vi "Compensate For Hit Position.vi"(8 "Primary channel":i8, 9 "Secondary hit time":u64, 10 "Secondary channel":i8, 11 "Primary hit time":u64) -> (2 "Secondary true hit time":u64, 3 "Primary true hit time":u64)   [LabVIEW 2016]
uses:
  Global Variables/Global Resolution.vi
panel:
  # "Calculates the actual muon hit time by compensating for the time it takes the photons to reach the SiPM"
  # "Leave primary hit time unwired to calculate secondary hit time and vice versa"
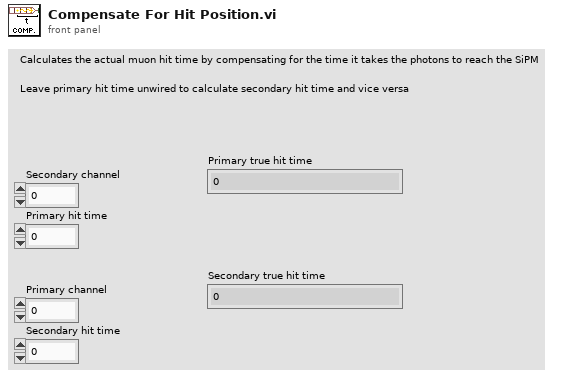
[diagram p1: front panel]
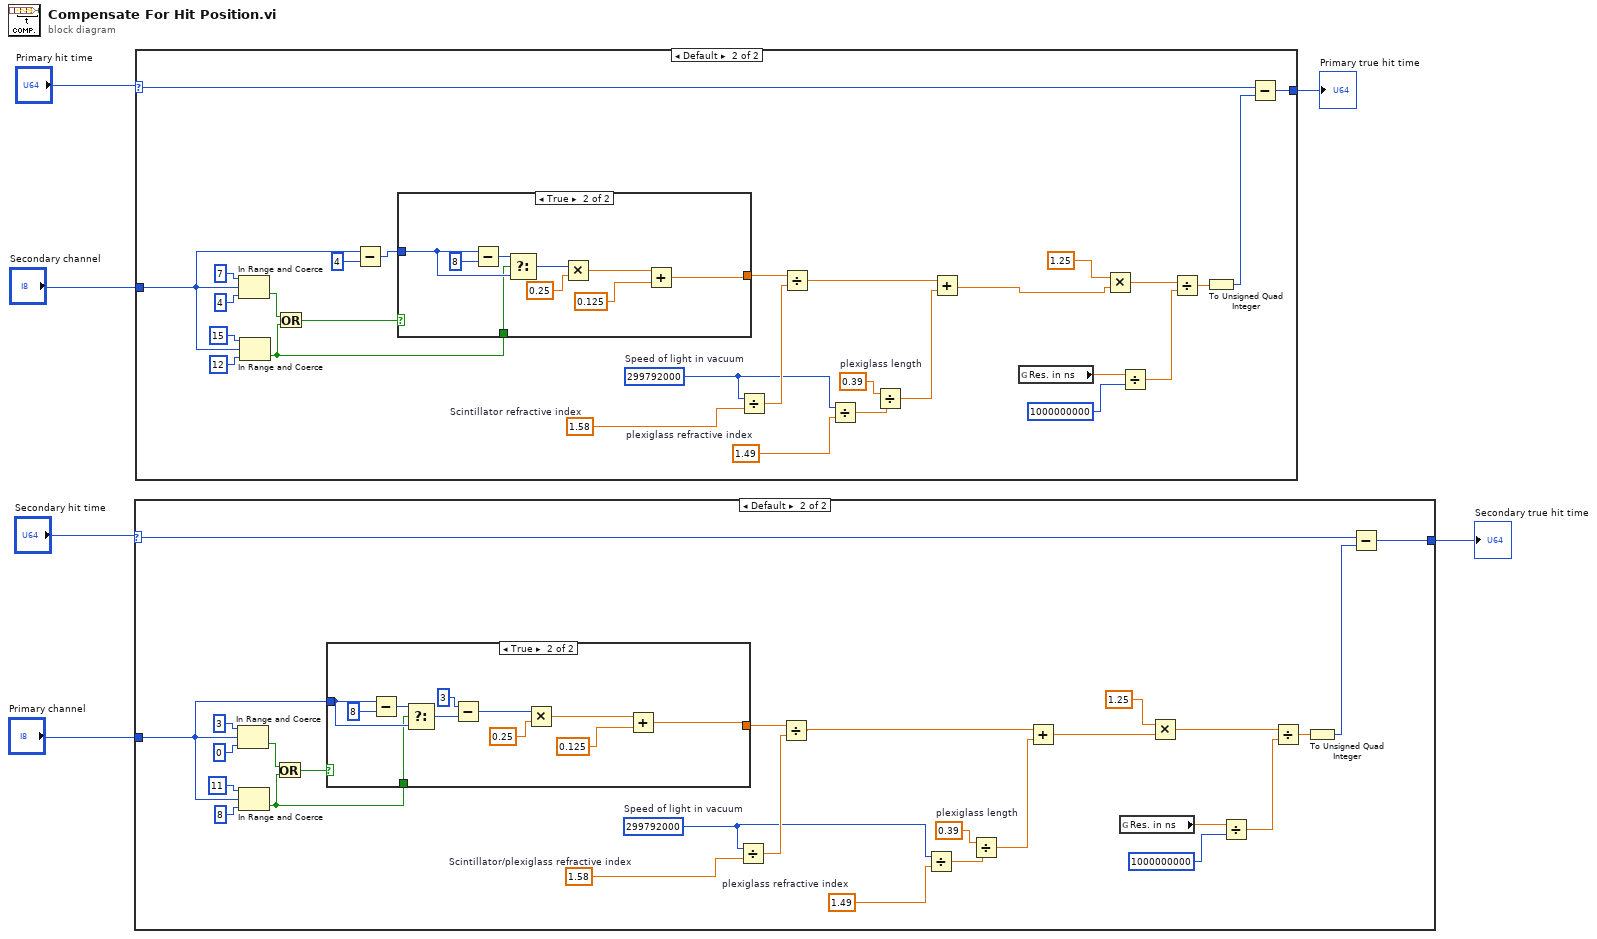
[diagram p0: block diagram]
diagram:
  n1 = case shown="Default" "Secondary hit time" {
    selector: "Secondary hit time" -> [w7 w18]
    tunnel: [w7 w19] -> w1
    tunnel: "Primary channel" -> [_ w17]
    frame 0 {
    }
    frame Default {
      w15 = 0.39  # plexiglass length
      w16 = 1.49  # plexiglass refractive index
      w11 = 299792000  # Speed of light in vacuum
      w34 = 1.58  # Scintillator/plexiglass refractive index
      n2 = In Range and Coerce(upper limit=3, x=w17, lower limit=0) -> (In Range?=w28:bool)  [unwired: 1 out]
      n3 = In Range and Coerce(upper limit=11, x=w17, lower limit=8) -> (In Range?=w27:bool)  [unwired: 1 out]
      n4 = Or(x=w28, y=w27) -> (x .or. y?=w29:bool)
      n5 = case shown="True" w29 {
        tunnel: w17 -> [_ w43]
        tunnel: w27 -> [_ w42]
        tunnel: [_ w35] -> w26
        frame False {
        }
        frame True {
          n6 = Subtract(x=w43, y=8) -> (x-y=w44:i32)
          n7 = Select(t=w44, s=w42, f=w43) -> (s? t:f=w38:i32)
          n8 = Subtract(x=3 ("y"), y=w38) -> (x-y=w40:i32)
          n9 = Multiply(x=w40, y=0.25) -> (x*y=w36:dbl)
          n10 = Add(x=w36, y=0.125) -> (x+y=w35:dbl)
        }
      }
      n11 = Divide(x=w11, y=w34) -> (x/y=w25:dbl)
      n12 = Divide(x=w26, y=w25) -> (x/y=w12:dbl)
      n13 = Divide(x=w11, y=w16) -> (x/y=w14:dbl)
      n14 = Divide(x=w15, y=w14) -> (x/y=w13:dbl)
      n15 = Add(x=w12, y=w13) -> (x+y=w10:dbl)
      n16 = global read "Global Resolution.vi" "Res. in ns"() -> (w22:ext)
      n17 = Multiply(x=1.25, y=w10) -> (x*y=w9:dbl)
      n18 = Divide(x=w22, y=1000000000) -> (x/y=w20:ext)
      n19 = Divide(x=w9, y=w20) -> (x/y=w23:ext)
      n20 = To Unsigned Quad Integer(1:w23) -> (0:w24:u64)
      n21 = Subtract(x=w18, y=w24) -> (x-y=w19:u64)
    }
  }
  "Secondary true hit time" <- w1
  n22 = case shown="Default" "Primary hit time" {
    selector: "Primary hit time" -> [w46 w56]
    tunnel: [w46 w60] -> w6
    tunnel: "Secondary channel" -> [_ w58]
    frame 0 {
    }
    frame Default {
      w53 = 0.39  # plexiglass length
      w54 = 1.49  # plexiglass refractive index
      w55 = 299792000  # Speed of light in vacuum
      w75 = 1.58  # Scintillator refractive index
      n23 = In Range and Coerce(upper limit=7, x=w58, lower limit=4) -> (In Range?=w69:bool)  [unwired: 1 out]
      n24 = In Range and Coerce(upper limit=15, x=w58, lower limit=12) -> (In Range?=w68:bool)  [unwired: 1 out]
      n25 = Or(x=w69, y=w68) -> (x .or. y?=w70:bool)
      n26 = Subtract(x=w58, y=4) -> (x-y=w57:i32)
      n27 = case shown="True" w70 {
        tunnel: w57 -> [_ w82]
        tunnel: w68 -> [_ w81]
        tunnel: [_ w77] -> w67
        frame False {
        }
        frame True {
          n28 = Subtract(x=w82, y=8) -> (x-y=w83:i32)
          n29 = Select(t=w83, s=w81, f=w82) -> (s? t:f=w80:i32)
          n30 = Multiply(x=w80, y=0.25) -> (x*y=w78:dbl)
          n31 = Add(x=w78, y=0.125) -> (x+y=w77:dbl)
        }
      }
      n32 = Divide(x=w55, y=w75) -> (x/y=w66:dbl)
      n33 = Divide(x=w67, y=w66) -> (x/y=w51:dbl)
      n34 = Divide(x=w55, y=w54) -> (x/y=w52:dbl)
      n35 = Divide(x=w53, y=w52) -> (x/y=w50:dbl)
      n36 = Add(x=w51, y=w50) -> (x+y=w47:dbl)
      n37 = global read "Global Resolution.vi" "Res. in ns"() -> (w63:ext)
      n38 = Multiply(x=1.25, y=w47) -> (x*y=w48:dbl)
      n39 = Divide(x=w63, y=1000000000) -> (x/y=w61:ext)
      n40 = Divide(x=w48, y=w61) -> (x/y=w64:ext)
      n41 = To Unsigned Quad Integer(1:w64) -> (0:w65:u64)
      n42 = Subtract(x=w56, y=w65) -> (x-y=w60:u64)
    }
  }
  "Primary true hit time" <- w6
